vi "Get GEA3 Serial Number.vi"(11 "Error In":errorcluster) -> (4 "GEA3 Serial Numbers":string[](array[string]), 15 "Error Out":errorcluster)   [LabVIEW 2023, in "GEA2_Toolkit.lvlib"]
uses:
  library/GEA2_Toolkit.lvlib
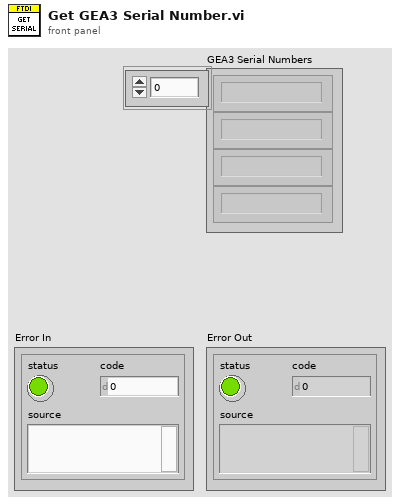
[diagram p1: front panel]
types:
  T1 = cluster{"Type":u32, "VID":string, "PID":string, "Serial Number":string, "Description":string}
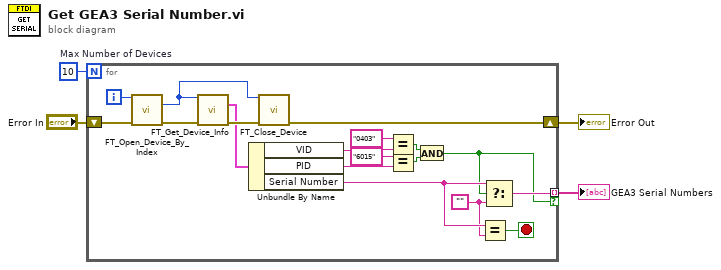
[diagram p0: block diagram]
diagram:
  w2 = 10  # Max Number of Devices
  n1 = for {
    N: w2 -> [_]
    shift-right: [w21] -> w3
    shift-left: "Error In" -> [w22]
    tunnel: [w7] -> w1 mode=indexing if=w6
    i -> [w17]
    stop <- w8 stop-if-true
    w5 = ""
    n2 = call "FT_Open_Device_By_Index.vi"("Device Index"=w17, "Error In"=w22) -> ("Handle"=w20:u32, "Error Out"=w19:errorcluster)  [unwired: 11 in, 1 out]
    n3 = call "FT_Get_Device_Info.vi"("Handle"=w20, "Error In"=w19) -> ("Device Information"=w16:T1, "Error Out"=w18:errorcluster)  [unwired: 11 in, 1 out]
    n4 = Unbundle By Name(w16) -> ("VID"=w15:string, "PID"=w14:string, "Serial Number"=w9:string)
    n5 = call "FT_Close_Device.vi"("Handle"=w20, "Error In"=w18) -> ("Error Out"=w21:errorcluster)  [unwired: 12 in, 1 out]
    n6 = Equal?(x="0403", y=w15) -> (x = y?=w11:bool)
    n7 = Equal?(x="6015", y=w14) -> (x = y?=w10:bool)
    n8 = And(x=w11, y=w10) -> (x .and. y?=w6:bool)
    n9 = Equal?(x=w9, y=w5) -> (x = y?=w8:bool)
    n10 = Select(t=w9, s=w6, f=w5) -> (s? t:f=w7:string)
  }
  "Error Out" <- w3
  "GEA3 Serial Numbers" <- w1
